vi "GetInputName.vi"(8 "error in (no error)":errorcluster, 10 "index":i32, 11 "session id in":i32) -> (0 "error out":errorcluster, 1 "InputName":string, 3 "session id out":i32)   [LabVIEW 2017, in "libonnx_wrapper.lvlib"]
doc: "/**\n * @brief Получить имя входа по индексу\n * \n * Каждому входу ONNX модели присвоено уникальное имя. Это имя необходимо\n * указывать при выполнении инференса. Функция копирует имя в предоставленный буфер.\n * \n * @param sessionId [IN] ID сессии\n * @param index [IN] Индекс входа (0-based, от 0 до GetInputCount-1)\n * @param buffer [OUT] Буфер для строки с именем (должен быть выделен в LabVIEW)\n * @param bufferSize [IN] Размер буфера в байтах (рекомендуется 256 или больше)\n * \n * @return int32: 0 при успешном копировании имени\n * @return int32: -1 если сессия не найдена, индекс неверен или буфер слишком мал\n * \n * @note Буфер должен быть выделен в LabVIEW перед вызовом\n * @note Имя завершается нулевым байтом ('\\0')\n */\nint GetInputName(int sessionId, int index, char* buffer, int bufferSize);"
uses:
  libonnx_wrapper.lvlib
panel:
  out "bufferSize":i32
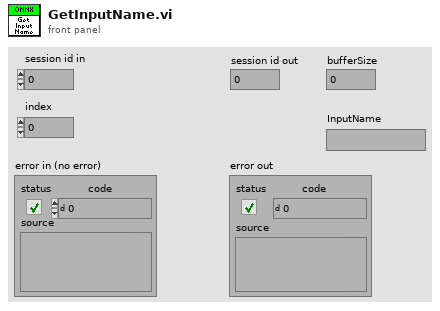
[diagram p1: front panel]
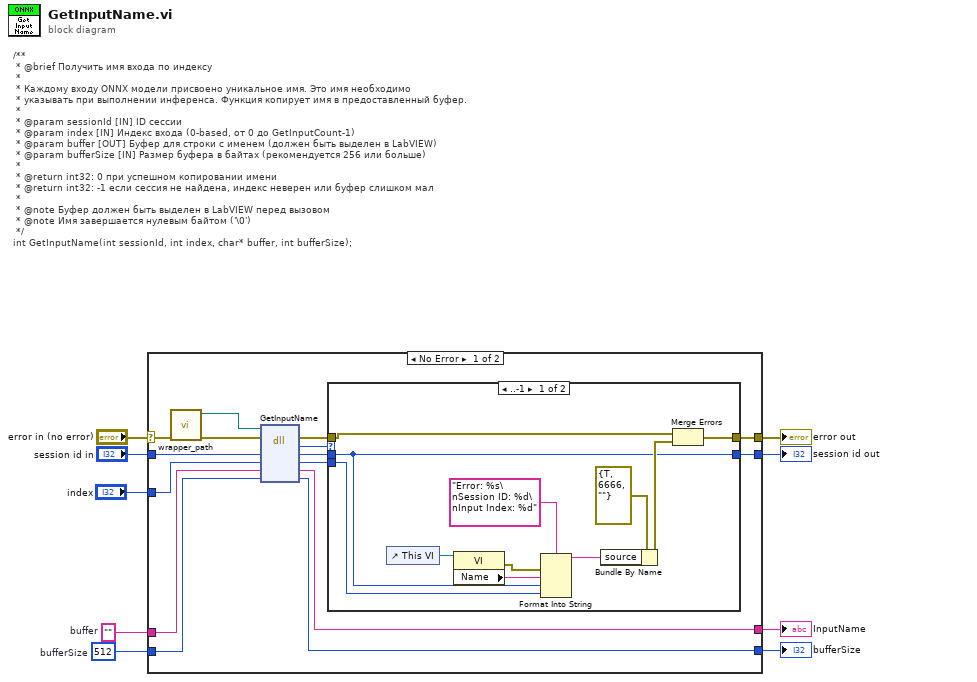
[diagram p0: block diagram]
diagram:
  w6 = 512  # bufferSize
  w8 = ""  # buffer
  # "/**\n * @brief Получить имя входа по индексу\n * \n * Каждому входу ONNX модели присвоено уникальное имя. Это имя необходимо\n * указывать при выполнении инференса. Функция копирует имя в предоставленный буфер.\n * \n * @param sessionId [IN] ID сессии\n * @param index [IN] Индекс входа (0-based, от 0 до GetInputCount-1)\n * @param buffer [OUT] Буфер для строки с именем (должен быть выделен в LabVIEW)\n * @param bufferSize [IN] Размер буфера в байтах (рекомендуется 256 или больше)\n * \n * @return int32: 0 при успешном копировании имени\n * @return int32: -1 если сессия не найдена, индекс неверен или буфер слишком мал\n * \n * @note Буфер должен быть выделен в LabVIEW перед вызовом\n * @note Имя завершается нулевым байтом ('\\0')\n */\nint GetInputName(int sessionId, int index, char* buffer, int bufferSize);"
  n1 = case shown="No Error" "error in (no error)" {
    selector: "error in (no error)" -> [w10 w39]
    tunnel: "index" -> [w24 _]
    tunnel: w8 -> [w23 _]
    tunnel: [w22 _] -> w7
    tunnel: w6 -> [w21 _]
    tunnel: "session id in" -> [w19 w38]
    tunnel: [w17 _] -> w4
    tunnel: [w13 w39] -> w3
    tunnel: [w12 w38] -> w2
    frame No Error {
      n2 = call "wrapper_path.vi"("error in (no error)"=w10) -> ("error out"=w18:errorcluster, "wrapper path"=w20:path)  [unwired: 9 in]
      n3 = dll-call lib="home/ivan/LabVIEWData/ONNX/Test/libonnx_wrapper/unix64/libonnx_wrapper.so" fn="GetInputName"(path in=w20, error in=w18, "sessionId"=w19, "index"=w24, "buffer"=w23, "bufferSize"=w21) -> (error out=w16:errorcluster, "return"=w15:i32, "sessionId"=w14:i32, "index"=w11:i32, "buffer"=w22:string, "bufferSize"=w17:i32)  [unwired: 1 in, 1 out]
      n4 = case shown="..-1" w15 {
        tunnel: w16 -> [w26 w37]
        tunnel: [w27 w37] -> w13
        tunnel: w14 -> [w28 w36]
        tunnel: [w28 w36] -> w12
        tunnel: w11 -> [w25 _]
        frame ..-1 {
          n5 = control-ref of="This VI"() -> (w32:refnum<vi>)
          n6 = property class="VI"(reference=w32) -> (error out=w29:errorcluster, "Name"=w31:string)  [unwired: 1 in, 1 out]
          n7 = Format Into String(format string="Error: %s\nSession ID: %d\nInput Index: %d", error in=w29, w31, w28, w25) -> (resulting string=w33:string)  [unwired: 1 in, 1 out]
          n8 = Bundle By Name(cluster=errorcluster {"status"=TRUE, "code"=6666, "source"=""} ("error out"), "source"=w33) -> (w34:errorcluster)
          n9 = Merge Errors(w26, w34) -> (w27:errorcluster)
        }
        frame 0.. {
        }
      }
    }
    frame Error {
    }
  }
  "error out" <- w3
  "session id out" <- w2
  "InputName" <- w7
  "bufferSize" <- w4
